vi "DSF.Shared.Configuration.Channel.New.vi"(8 "error in (no error)":errorcluster, 10 "channel parameters":T1 {"VS channel ref" format="%x"}, 11 "Channel Configuration type":refnum<class "DSF.Shared.Configuration.Channel.lvclass">) -> (0 "error out":errorcluster, 3 "Channel Configuration out":refnum<class "DSF.Shared.Configuration.Channel.lvclass">)   [LabVIEW 2016, in "DSF.Shared.lvlib" / "DSF.Shared.Configuration.Channel.lvclass"]
uses:
  DSF.Shared.Configuration.Channel.lvclass
  DSF.Shared.Configuration.Channel.Parameters.ctl
  Typedefs/DSF.Shared.Typedefs.Data Type.ctl
  DSF.Shared.Configuration.Channel.lvclass/DSF.Shared.Configuration.Channel.ctl
  DSF.Shared.lvlib
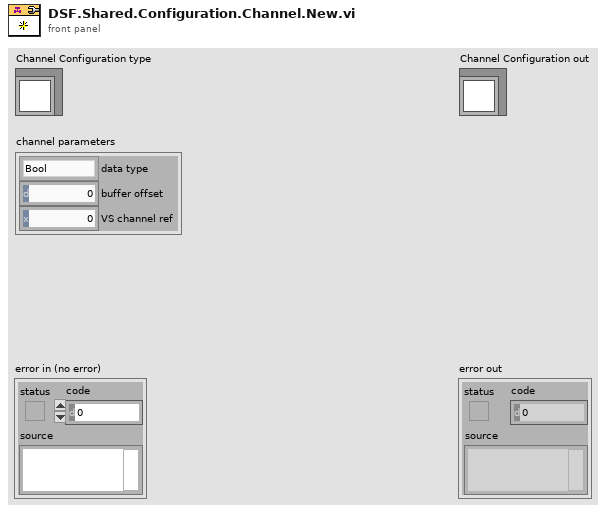
[diagram p1: front panel]
types:
  T1 = typedef "DSF.Shared.lvlib/DSF.Shared.Configuration.Channel.lvclass/DSF.Shared.Configuration.Channel.Parameters.ctl" = cluster{"data type":T2, "buffer offset":u64, "VS channel ref":u64}
  T2 = typedef "DSF.Shared.lvlib/DSF.Shared.Typedefs.Data Type.ctl" = enum8{"Bool", "SGL", "DBL", "I8", "I16", "I32", "I64", "U8", "U16", "U32", "U64"}
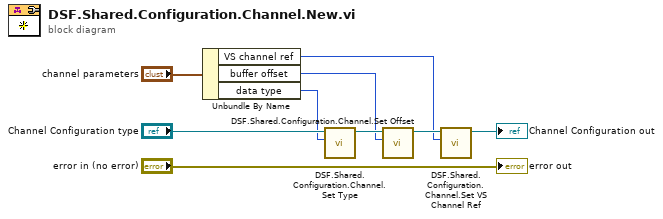
[diagram p0: block diagram]
diagram:
  n1 = Unbundle By Name("channel parameters") -> ("VS channel ref"=w4:u64, "buffer offset"=w3:u64, "data type"=w2:T2)
  n2 = call "DSF.Shared.Configuration.Channel.Set Type.vi"("data type"=w2, "Channel Configuration in"="Channel Configuration type") -> ("Channel Configuration out"=w7:refnum<class "DSF.Shared.Configuration.Channel.lvclass">)  [unwired: 9 in]
  n3 = call "DSF.Shared.Configuration.Channel.Set Offset.vi"("buffer offset"=w3, "Channel Configuration in"=w7) -> ("Channel Configuration out"=w6:refnum<class "DSF.Shared.Configuration.Channel.lvclass">)  [unwired: 9 in]
  n4 = call "DSF.Shared.Configuration.Channel.Set VS Channel Ref.vi"("VS channel ref"=w4, "Channel Configuration in"=w6) -> ("Channel Configuration out"=→"Channel Configuration out":refnum<class "DSF.Shared.Configuration.Channel.lvclass">)  [unwired: 9 in]
  "error out" <- "error in (no error)"
